vi "Format Event Timing Measurements into Table.vi"(11 "Measurements":T1[](array[typedef])) -> (3 "Table":string[][](array[string]))   [LabVIEW 2015, in "Engine Simulation Toolkit System Explorer.lvlib"]
uses:
  Engine Simulation Toolkit System Explorer.lvlib
  Event Timing Measurement.ctl
  Polarity.ctl
  Shared/Constants and GUIDs.vi
  Shared/Engine Simulation Toolkit Shared.lvlib
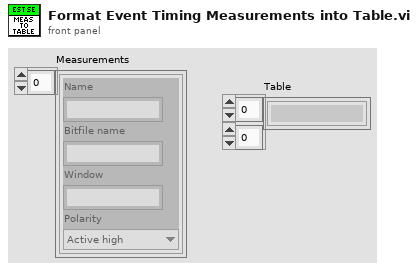
[diagram p1: front panel]
types:
  T1 = typedef "Engine Simulation Toolkit System Explorer.lvlib/Event Timing Measurement.ctl" = cluster{"Name":string, "Bitfile name":string, "Window":string, "Polarity":T2}
  T2 = typedef "Engine Simulation Toolkit System Explorer.lvlib/Polarity.ctl" = enum16{"Active low", "Active high"}
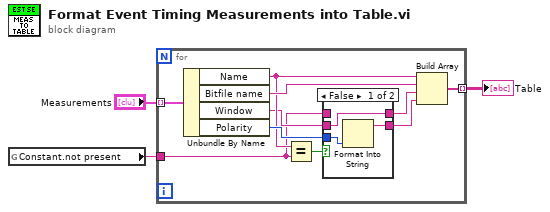
[diagram p0: block diagram]
diagram:
  n1 = global read "Constants and GUIDs.vi" "Constant.not present"() -> (w1:string)
  n2 = for {
    tunnel: "Measurements" -> [w13] mode=indexing
    tunnel: [w12] -> w2 mode=indexing
    tunnel: w1 -> [w4]
    n3 = Unbundle By Name(w13) -> ("Name"=w8:string, "Bitfile name"=w11:string, "Window"=w5:string, "Polarity"=w10:T2)
    n4 = Equal?(x=w8, y=w4) -> (x = y?=w7:bool)
    n5 = case shown="False" w7 {
      tunnel: w10 -> [w16 _]
      tunnel: [w15 w17] -> w9
      tunnel: [w14 w17] -> w6
      tunnel: w5 -> [w14 _]
      tunnel: w4 -> [_ w17]
      frame False {
        n6 = Format Into String(w16) -> (resulting string=w15:string)  [unwired: 3 in, 1 out]
      }
      frame True {
      }
    }
    n7 = Build Array(w8, w11, w6, w9) -> (w12:string[])
  }
  "Table" <- w2
